vi "ColortoHSV.vi"(8 "error in (no error)":errorcluster, 11 "Color Box":u32(colorbox)) -> (0 "error out":errorcluster, 1 "Value (0-255)":u8, 2 "Saturation (0-255)":u8=1, 3 "Hue (0-180)":u8)   [LabVIEW 2014, in "QwaveSys RPi Training Library.lvlib"]
uses:
  <vilib>/Q-Wave Systems/QwaveSys RPi Package 2.0/Addons/QwaveSys RPi Training Library.lvlib
panel:
  out "B":u8
  out "G":u8
  out "R":u8
  out "Color Box Out":u32(colorbox)
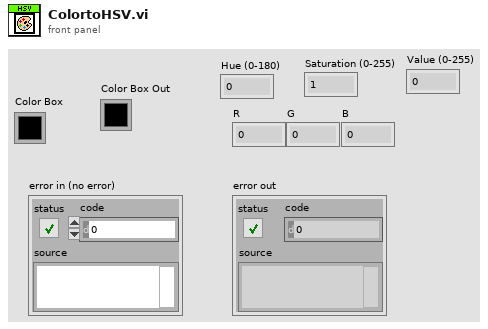
[diagram p1: front panel]
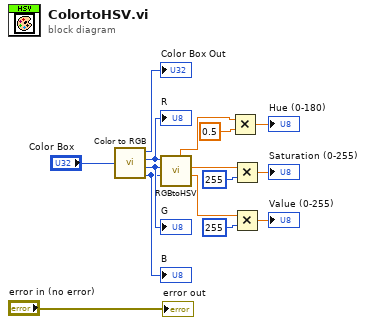
[diagram p0: block diagram]
diagram:
  n1 = call <vilib>:"Color to RGB.vi"("Color"="Color Box") -> ("Resolved Color"=→"Color Box Out":u32, "R"=w13:u8, "G"=w12:u8, "B"=w11:u8)
  "R" <- w13
  "G" <- w12
  "B" <- w11
  n2 = call <vilib>:"RGBtoHSV.vi"("Blue"=w11, "Green"=w12, "Red"=w13) -> ("Value"=w4:dbl, "Saturation"=w6:dbl, "Hue (0-360)"=w10:dbl)  [unwired: 5 in, 1 out]
  n3 = Multiply(x=w10, y=0.5) -> (x*y=→"Hue (0-180)":dbl)
  n4 = Multiply(x=w6, y=u8 255) -> (x*y=→"Saturation (0-255)":dbl)
  n5 = Multiply(x=w4, y=u8 255) -> (x*y=→"Value (0-255)":dbl)
  "error out" <- "error in (no error)"
